vi "OxITC503 _Control_ Local-remote.vi"(2 "error in":errorcluster, 3 "Control Status":T1(ring), 4 "VISA session":refnum<visa-resource-name>) -> (0 "error out (no error)":errorcluster, 1 "VISA session":refnum<visa-resource-name>)   [LabVIEW 2013]
doc: "Sets ITC503 into LOCAL or REMOTE and determines whether the LOC/REM buttom is LOCKED or active."
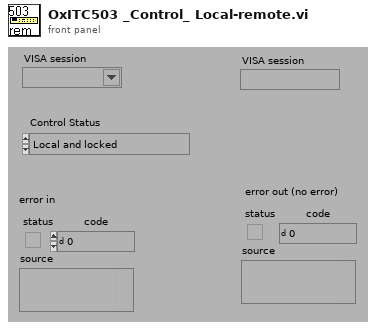
[diagram p1: front panel]
types:
  T1 = enum16{"Local and locked", "Remote and Locked", "Local and unlocked", "Remote and Unlocked"}
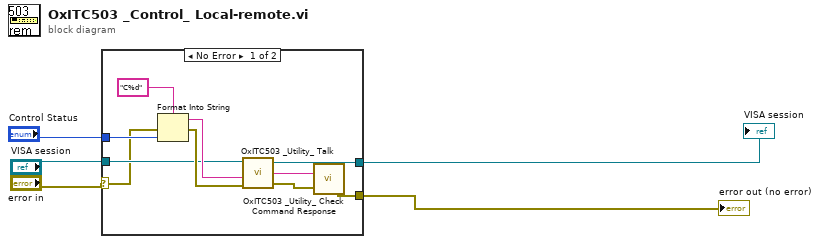
[diagram p0: block diagram]
diagram:
  n1 = case shown="No Error" "error in" {
    selector: "error in" -> [w6 w16]
    tunnel: "Control Status" -> [w13 _]
    tunnel: [w11 w17] -> w4
    tunnel: "VISA session" -> [w10 w17]
    tunnel: [w7 w16] -> w2
    frame No Error {
      n2 = Format Into String(format string="C%d" ("Format String"), error in=w6, w13) -> (resulting string=w14:string, error out=w15:errorcluster)  [unwired: 1 in]
      n3 = call "OxITC503 _Utility_ Talk.vi"("VISA session"=w10, "Command"=w14, "error in (no error)"=w15) -> ("VISA session"=w11:refnum<visa-resource-name>, "read buffer"=w9:string, "error out (no error)"=w8:errorcluster)  [unwired: 2 in]
      n4 = call "OxITC503 _Utility_ Check Command Response.vi"("error in"=w8, "read buffer"=w9) -> ("error out (no error)"=w7:errorcluster)  [unwired: 1 out]
    }
    frame Error {
    }
  }
  "error out (no error)" <- w2
  "VISA session" <- w4
